vi "CreateSnapshot.vi"(8 "Error In":errorcluster, 11 "Snapshot Path (*.json)":path) -> (0 "Error Out":errorcluster, 3 "SystemSnapshot":T1={"FeedURLs"=["https://download.ni.com/support/nipkg/products/ni-t/ni-teststand-2020/20.0/released"], "Packages"=[]})   [LabVIEW 2019, in "CEPM.lvlib"]
uses:
  CEPM.lvlib
  <vilib>/National Instruments/NIPM API (Beta)/NIPM_API.lvlib
  Typedefs/SystemSnapshot.ctl
  96cc1ed3-5d77-4aac-821a-2495f093d2c6.vi
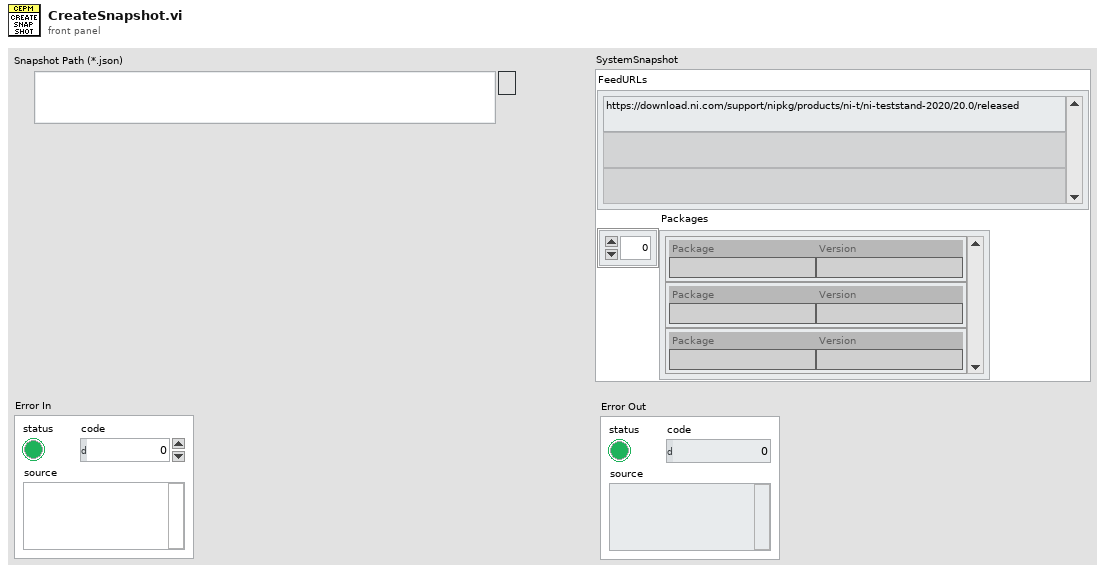
[diagram p1: front panel]
types:
  T1 = typedef "CEPM.lvlib/SystemSnapshot.ctl" = cluster{"FeedURLs":string[], "Packages":cluster{"Package":string, "Version":string}[]}
  T2 = typedef "NIPM_API.lvlib/feed.ctl" = cluster{"Name":string, "URI":string}
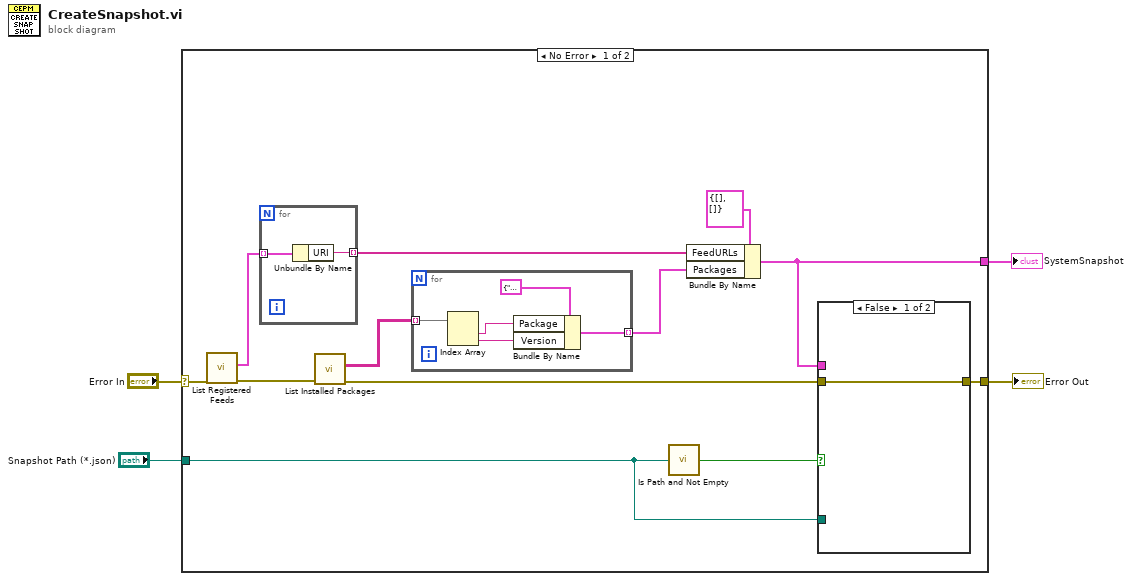
[diagram p0: block diagram]
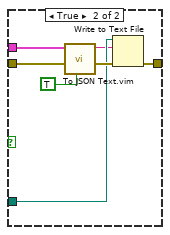
[diagram p2: hidden frame]
diagram:
  n1 = case shown="No Error" "Error In" {
    selector: "Error In" -> [w16 w32]
    tunnel: [w7 w32] -> w3
    tunnel: "Snapshot Path (*.json)" -> [w6 _]
    tunnel: [w8 _] -> w1
    frame No Error {
      n2 = call <vilib>:"List Registered Feeds.vi"("error in"=w16) -> ("error out"=w14:errorcluster, "registered feeds"=w15:T2[])  [unwired: 9 in]
      n3 = for {
        tunnel: w15 -> [w31] mode=indexing
        tunnel: [w30] -> w10 mode=indexing
        n4 = Unbundle By Name(w31) -> ("URI"=w30:string)
      }
      n5 = call <vilib>:"List Installed Packages.vi"("error in"=w14) -> ("error out"=w12:errorcluster, "installed packages"=w13:string[][])  [unwired: 9 in]
      n6 = for {
        tunnel: w13 -> [w29] mode=indexing
        tunnel: [w25] -> w9 mode=indexing
        n7 = Index Array(array=w29) -> (element #1=w27:string, element #2=w26:string)  [unwired: 2 in]
        n8 = Bundle By Name(cluster=cluster{"Package":string, "Version":string} {"Package"="", "Version"=""} ("PackageMeta"), "Package"=w27, "Version"=w26) -> (w25:cluster{"Package":string, "Version":string})
      }
      n9 = call <vilib>:"Is Path and Not Empty.vi"("path"=w6) -> ("Is Path and Not Empty?"=w5:bool)  [unwired: 4 in]
      n10 = Bundle By Name(cluster=T1 {"FeedURLs"=[], "Packages"=[]} ("SystemSnapshot"), "FeedURLs"=w10, "Packages"=w9) -> (w8:T1)
      n11 = case shown="False" w5 {
        tunnel: w12 -> [w17 w24]
        tunnel: w8 -> [_ w22]
        tunnel: [w17 w20] -> w7
        tunnel: w6 -> [_ w19]
        frame False {
        }
        frame True {
          n12 = call "To JSON Text.vim"("Pretty Print?"=TRUE, "error in (no error)"=w24, "Anything"=w22) -> ("error out"=w23:errorcluster, "<JSON>"=w18:string)  [unwired: 7 in]
          n13 = Write to Text File(file (use dialog)=w19, text=w18, error in=w23) -> (error out=w20:errorcluster)  [unwired: 1 in, 2 out]
        }
      }
    }
    frame Error {
    }
  }
  "Error Out" <- w3
  "SystemSnapshot" <- w1
